vi "RS触发器（反馈节点）.vi"(8 "R":bool, 11 "S":bool) -> (3 "Q":bool)   [LabVIEW 2012, in "触发器.lvlib"]
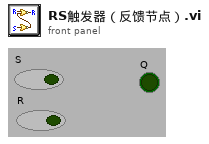
[diagram p1: front panel]
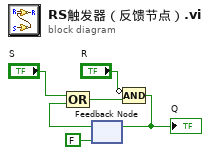
[diagram p0: block diagram]
diagram:
  n1 = feedback #1(FALSE) -> (w1:bool)
  n2 = Compound Arithmetic op=OR ("OR")("S", w1) -> (w6:bool)
  n3 = Compound Arithmetic op=AND ("AND")(invert "R", w6) -> (w5:bool)
  "Q" <- w5
  n4 = feedback-in #1(w5) -> ()
